vi "Test Count.vi"(8 "error in (no error)":errorcluster, 10 "Test Log":i32(ring) items=["Baseboard", "SubModule1", "SubModule2"], 11 "Instrument Handle In":i32(ring)) -> (0 "error out":errorcluster, 2 "Number of Reports":i32 caption="Number of Errors", 3 "Instrument Handle Out":i32(ring))   [LabVIEW 8.6, in "ZTScopeM.lvlib"]
doc: "Query the number of self test report entries for the specified log."
uses:
  ZTScopeM.lvlib
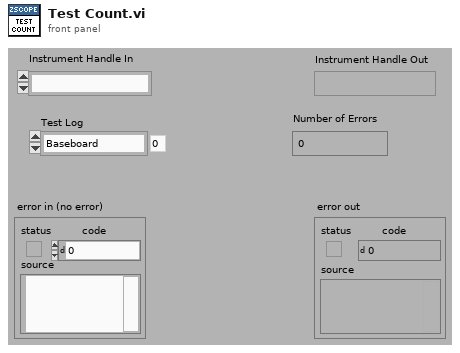
[diagram p1: front panel]
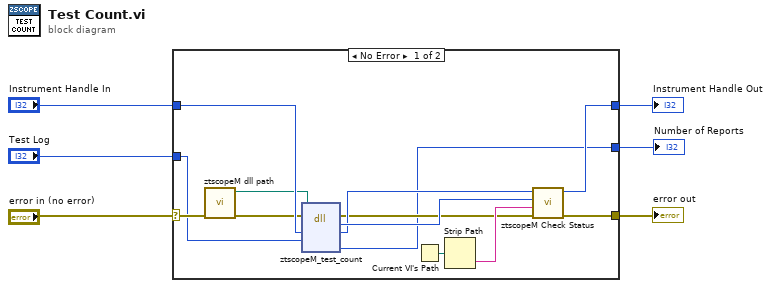
[diagram p0: block diagram]
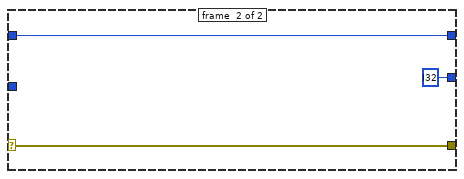
[diagram p2: hidden frame]
diagram:
  n1 = case shown="No Error" "error in (no error)" {
    selector: "error in (no error)" -> [w12 w22]
    tunnel: [w13 w22] -> w5
    tunnel: "Instrument Handle In" -> [w18 w21]
    tunnel: [w14 w21] -> w3
    tunnel: "Test Log" -> [w8 _]
    tunnel: [w7 i32 ? ("Number of Errors")] -> w1
    frame #0 {
      n2 = call "ztscopeM dll path.vi"("error in (no error)"=w12) -> ("error out"=w10:errorcluster, "<instrument>.dll path"=w11:path)  [unwired: 9 in]
      n3 = dll-call lib="C:/Program Files (x86)/National Instruments/LabVIEW 2013/instr.lib/ztscopem/ztscopeM.dll" fn="ztscopeM_test_count"(path in=w11, error in=w10, "Instrument Handle"=w18, "Test Log"=w8) -> (error out=w9:errorcluster, "Status"=w16:i32, "Instrument Handle"=w15:i32, "Number of Errors"=w7:i32)  [unwired: 3 in, 1 out]
      n4 = Current VI's Path() -> (path=w19:path)
      n5 = Strip Path(path=w19) -> (name=w17:string)  [unwired: 1 out]
      n6 = call "ztscopeM Check Status.vi"("error in"=w9, "name of VI"=w17, "status (return code)"=w16, "instrument handle in"=w15) -> ("error out"=w13:errorcluster, "instrument handle out"=w14:i32)  [unwired: 2 in]
    }
    frame #1 {
    }
  }
  "error out" <- w5
  "Instrument Handle Out" <- w3
  "Number of Reports" <- w1
